vi "Autopatcher Daemon.vi"(0 "Controls":T8, 1 "Break in Thr [MOhm]":refnum<vi>, 2 "Detection Thr [%]":refnum<vi>, 3 "Disengage Target":refnum<vi>, 4 "Manipulator Dynamics":refnum<vi>, 5 "Unblockage Parameters":T7, 6 "Sensed Resistance Levels":T4, 7 "Error In":errorcluster, 8 "Signals":T9, 9 "Pressure Controls":T11, 10 "Holding Potential Controls":T2, 11 "Autotune Gain":T3, 12 "Calibration levels":T6, 13 "Manipulator Controllers":T10, 14 "Capacitance Compensation":refnum<vi>, 15 "Test and Offset Controls":T5, 16 "Dialog Indicator":refnum<vi>, 17 "Seal Dynamics":T1, 18 "Reset":refnum<vi>, 19 "Manipulator Transformation Matrix":refnum<vi>, 20 "State":refnum<vi>) -> (27 "Error Out":errorcluster)   [LabVIEW 2012, in "Autopatcher Daemon.lvlib"]
uses:
  Autopatcher Daemon.lvlib
  <vilib>/Analysis/Matrix/Datatypes/RealMatrix.ctl
  State.ctl
  <vilib>/Analysis/Matrix/NI_Matrix.lvlib
panel:
  out "Abort":refnum<vi>
  out "Exit":bool
  in  "Period":u32=100
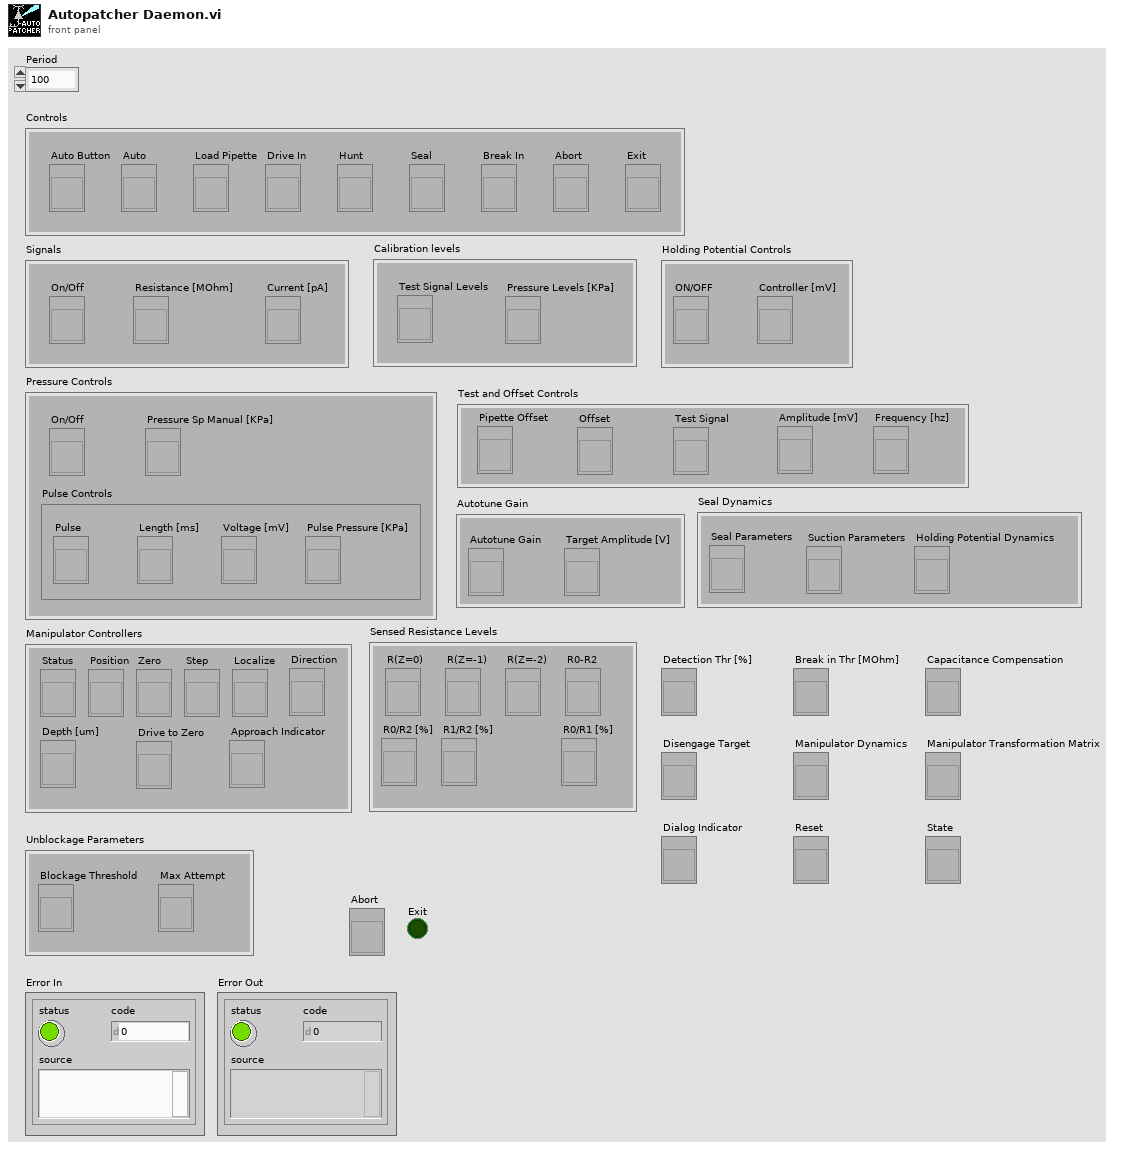
[diagram p1: front panel]
types:
  T1 = cluster{"Suction Parameters":refnum<vi>, "Holding Potential Dynamics":refnum<vi>, "Seal Parameters":refnum<vi>}
  T2 = cluster{"ON/OFF":refnum<vi>, "Controller [mV]":refnum<vi>}
  T3 = cluster{"Autotune Gain":refnum<vi>, "Target Amplitude [V]":refnum<vi>}
  T4 = cluster{"R(Z=0)":refnum<vi>, "R(Z=-1)":refnum<vi>, "R(Z=-2)":refnum<vi>, "R0-R2":refnum<vi>, "R0/R2 [%]":refnum<vi>, "R1/R2 [%]":refnum<vi>, "R0/R1 [%]":refnum<vi>}
  T5 = cluster{"Pipette Offset":refnum<vi>, "Offset":refnum<vi>, "Test Signal":refnum<vi>, "Amplitude [mV]":refnum<vi>, "Frequency [hz]":refnum<vi>}
  T6 = cluster{"Test Signal Levels":refnum<vi>, "Pressure Levels [KPa]":refnum<vi>}
  T7 = cluster{"Blockage Threshold":refnum<vi>, "Max Attempt":refnum<vi>}
  T8 = cluster{"Load Pipette":refnum<vi>, "Drive In":refnum<vi>, "Hunt":refnum<vi>, "Seal":refnum<vi>, "Break In":refnum<vi>, "Abort":refnum<vi>, "Exit":refnum<vi>, "Auto":refnum<vi>, "Auto Button":refnum<vi>}
  T9 = cluster{"On/Off":refnum<vi>, "Resistance [MOhm]":refnum<vi>, "Current [pA]":refnum<vi>}
  T10 = cluster{"Status":refnum<vi>, "Position":refnum<vi>, "Zero":refnum<vi>, "Step":refnum<vi>, "Localize":refnum<vi>, "Approach Indicator":refnum<vi>, "Depth [um]":refnum<vi>, "Drive to Zero":refnum<vi>, "Direction":refnum<vi>}
  T11 = cluster{"On/Off":refnum<vi>, "Pulse Controls":cluster{"Pulse":refnum<vi>, "Length [ms]":refnum<vi>, "Voltage [mV]":refnum<vi>, "Pulse Pressure [KPa]":refnum<vi>}, "Pressure Sp Manual [KPa]":refnum<vi>}
  T12 = typedef "State.ctl" = enum16{"READY", "LOAD", "LOCALIZATION", "HUNTING", "SEAL", "BREAKIN", "WCR", "ALIGN", "APPROACH", "TARGETING"}
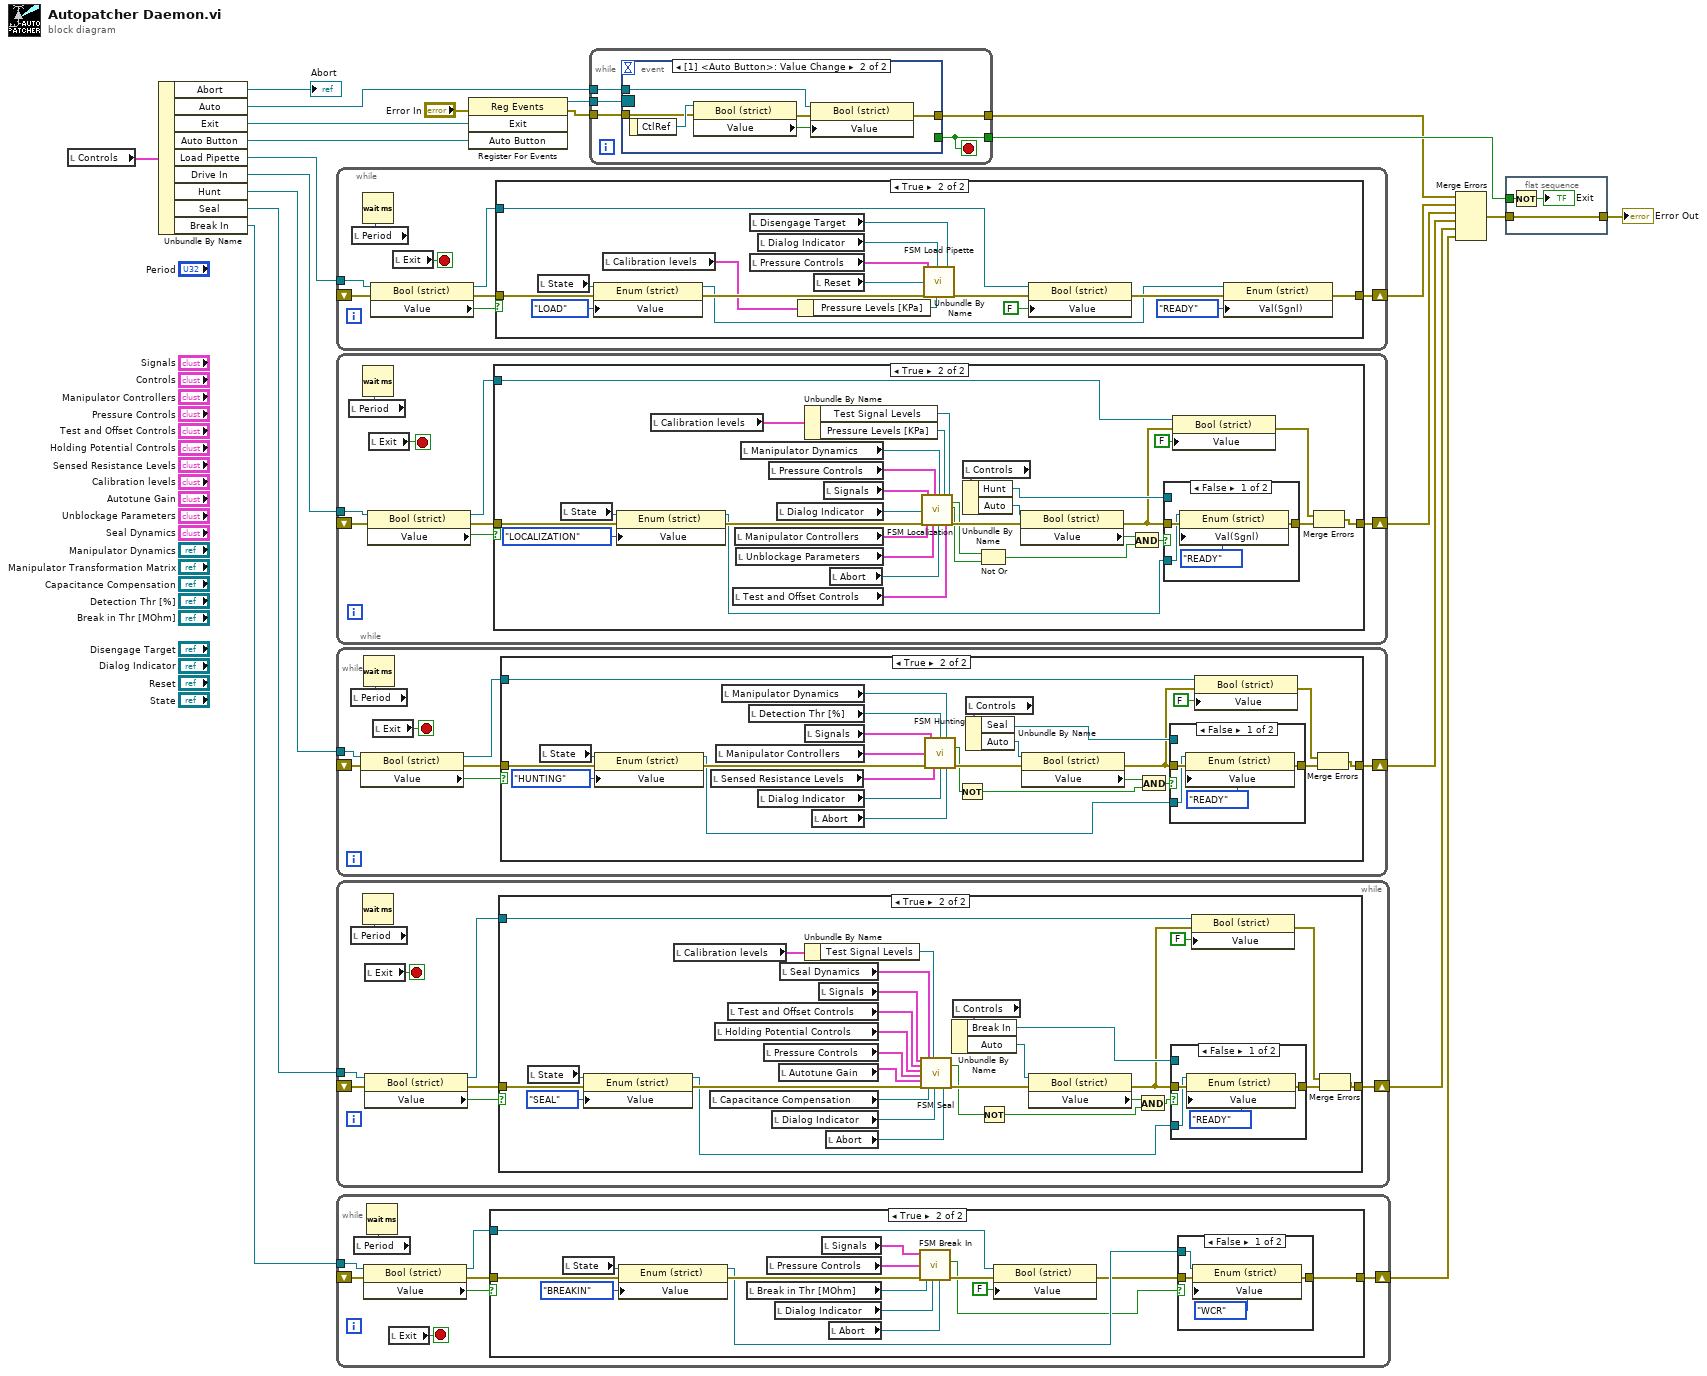
[diagram p0: block diagram]
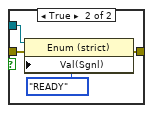
[diagram p3: hidden frame]
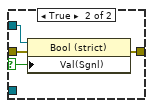
[diagram p5: hidden frame]
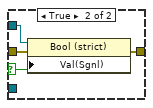
[diagram p7: hidden frame]
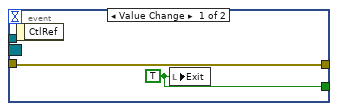
[diagram p8: hidden frame]
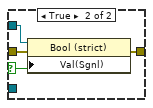
[diagram p10: hidden frame]
diagram:
  n1 = local read "Controls"() -> (w11:T8)
  n2 = Unbundle By Name(w11) -> ("Abort"=→"Abort":refnum<vi>, "Auto"=w3:refnum<vi>, "Exit"=w6:refnum<vi>, "Auto Button"=w5:refnum<vi>, "Load Pipette"=w16:refnum<vi>, "Drive In"=w15:refnum<vi>, "Hunt"=w13:refnum<vi>, "Seal"=w12:refnum<vi>, "Break In"=w10:refnum<vi>)
  n3 = while {
    tunnel: w16 -> [w30]
    shift-right: [w25] -> w21
    shift-left: _ -> [w23]
    stop <- w26 stop-if-true
    n4 = local read "Period"() -> (w27:u32)
    n5 = Wait (ms)(milliseconds to wait=w27) -> ()  [unwired: 1 out]
    n6 = property class="Bool (strict)"(reference=w30, error in=w23) -> (reference out=w24:refnum<vi>, error out=w28:errorcluster, "Value"=w29:bool)
    n7 = local read "Exit"() -> (w26:bool)
    n8 = case shown="True" w29 {
      tunnel: w28 -> [w31 w35]
      tunnel: [w31 w41] -> w25
      tunnel: w24 -> [_ w39]
      frame False {
      }
      frame True {
        n9 = local read "State"() -> (w38:refnum<vi>)
        n10 = property class="Enum (strict)"(reference=w38, error in=w35, "Value"=State."LOAD") -> (reference out=w34:refnum<vi>, error out=w36:errorcluster)
        n11 = local read "Calibration levels"() -> (w32:T6)
        n12 = local read "Disengage Target"() -> (w46:refnum<vi>)
        n13 = local read "Pressure Controls"() -> (w48:T11)
        n14 = local read "Dialog Indicator"() -> (w47:refnum<vi>)
        n15 = Unbundle By Name(w32) -> ("Pressure Levels [KPa]"=w33:refnum<vi>)
        n16 = local read "Reset"() -> (w45:refnum<vi>)
        n17 = call "FSM Load Pipette.vi"("Dialog Indicator"=w47, "Pressure Controls"=w48, "Reset"=w45, "error in (no error)"=w36, "Disengage Target"=w46, "Pressure Levels [KPa]"=w33) -> ("error out"=w40:errorcluster)  [unwired: 13 in]
        n18 = property class="Bool (strict)"(reference=w39, error in=w40, "Value"=FALSE) -> (error out=w42:errorcluster)  [unwired: 1 out]
        n19 = property class="Enum (strict)"(reference=w34, error in=w42, "Val(Sgnl)"=State."READY" ("Value")) -> (error out=w41:errorcluster)  [unwired: 1 out]
      }
    }
  }
  n20 = while {
    tunnel: w15 -> [w56]
    shift-right: [w50] -> w20
    shift-left: _ -> [w49]
    stop <- w52 stop-if-true
    n21 = local read "Period"() -> (w53:u32)
    n22 = Wait (ms)(milliseconds to wait=w53) -> ()  [unwired: 1 out]
    n23 = property class="Bool (strict)"(reference=w56, error in=w49) -> (reference out=w51:refnum<vi>, error out=w54:errorcluster, "Value"=w55:bool)
    n24 = local read "Exit"() -> (w52:bool)
    n25 = case shown="True" w55 {
      tunnel: w54 -> [w57 w65]
      tunnel: [w57 w71] -> w50
      tunnel: w51 -> [_ w72]
      frame False {
      }
      frame True {
        n26 = local read "State"() -> (w67:refnum<vi>)
        n27 = property class="Enum (strict)"(reference=w67, error in=w65, "Value"=State."LOCALIZATION") -> (reference out=w61:refnum<vi>, error out=w66:errorcluster)
        n28 = local read "Calibration levels"() -> (w82:T6)
        n29 = local read "Test and Offset Controls"() -> (w80:T5)
        n30 = local read "Manipulator Controllers"() -> (w87:T10)
        n31 = local read "Unblockage Parameters"() -> (w83:T7)
        n32 = local read "Manipulator Dynamics"() -> (w88:refnum<vi>)
        n33 = local read "Pressure Controls"() -> (w86:T11)
        n34 = local read "Dialog Indicator"() -> (w79:refnum<vi>)
        n35 = Unbundle By Name(w82) -> ("Test Signal Levels"=w78:refnum<vi>, "Pressure Levels [KPa]"=w81:refnum<vi>)
        n36 = local read "Signals"() -> (w85:T9)
        n37 = local read "Abort"() -> (w84:refnum<vi>)
        n38 = call "FSM Localization.vi"("Signals"=w85, "Pressure Controls"=w86, "Dialog Indicator"=w79, "error in (no error)"=w66, "Manipulator Dynamics"=w88, "Unblockage Parameters"=w83, "Pressure Levels [KPa]"=w81, "Test and Offset Controls"=w80, "Test Signal Levels"=w78, "Manipulator Controllers"=w87, "Abort"=w84) -> ("Aborted"=w59:bool, "Blocked"=w60:bool, "error out"=w75:errorcluster)  [unwired: 6 in]
        n39 = local read "Controls"() -> (w76:T8)
        n40 = Unbundle By Name(w76) -> ("Hunt"=w74:refnum<vi>, "Auto"=w77:refnum<vi>)
        n41 = Not Or(1:w60, 2:w59) -> (0:w58:bool)
        n42 = property class="Bool (strict)"(reference=w77, error in=w75) -> (error out=w64:errorcluster, "Value"=w62:bool)  [unwired: 1 out]
        n43 = And(x=w62, y=w58) -> (x .and. y?=w63:bool)
        n44 = case shown="False" w63 {
          selector: w63 -> [_ w94]
          tunnel: w64 -> [w92 w96]
          tunnel: w74 -> [_ w95]
          tunnel: [w91 w93] -> w70
          tunnel: w61 -> [w90 _]
          frame False {
            n45 = property class="Enum (strict)"(reference=w90, error in=w92, "Val(Sgnl)"=State."READY" ("Value")) -> (error out=w91:errorcluster)  [unwired: 1 out]
          }
          frame True {
            n46 = property class="Bool (strict)"(reference=w95, error in=w96, "Val(Sgnl)"=w94) -> (error out=w93:errorcluster)  [unwired: 1 out]
          }
        }
        n47 = property class="Bool (strict)"(reference=w72, error in=w64, "Value"=FALSE) -> (error out=w69:errorcluster)  [unwired: 1 out]
        n48 = Merge Errors(w69, w70) -> (w71:errorcluster)
      }
    }
  }
  n49 = while {
    tunnel: w13 -> [w104]
    shift-right: [w98] -> w9
    shift-left: _ -> [w97]
    stop <- w102 stop-if-true
    n50 = local read "Period"() -> (w100:u32)
    n51 = property class="Bool (strict)"(reference=w104, error in=w97) -> (reference out=w99:refnum<vi>, error out=w101:errorcluster, "Value"=w103:bool)
    n52 = Wait (ms)(milliseconds to wait=w100) -> ()  [unwired: 1 out]
    n53 = local read "Exit"() -> (w102:bool)
    n54 = case shown="True" w103 {
      tunnel: w101 -> [w105 w113]
      tunnel: [w105 w117] -> w98
      tunnel: w99 -> [_ w124]
      frame False {
      }
      frame True {
        n55 = local read "State"() -> (w115:refnum<vi>)
        n56 = property class="Enum (strict)"(reference=w115, error in=w113, "Value"=State."HUNTING") -> (reference out=w106:refnum<vi>, error out=w114:errorcluster)
        n57 = local read "Sensed Resistance Levels"() -> (w126:T4)
        n58 = local read "Manipulator Controllers"() -> (w131:T10)
        n59 = local read "Manipulator Dynamics"() -> (w129:refnum<vi>)
        n60 = local read "Detection Thr [%]"() -> (w127:refnum<vi>)
        n61 = local read "Dialog Indicator"() -> (w128:refnum<vi>)
        n62 = local read "Signals"() -> (w130:T9)
        n63 = local read "Abort"() -> (w107:refnum<vi>)
        n64 = call "FSM Hunting.vi"("Signals"=w130, "Detection Thr [%]"=w127, "Manipulator Dynamics"=w129, "Manipulator Controllers"=w131, "Sensed Resistance Levels"=w126, "error in (no error)"=w114, "Dialog Indicator"=w128, "Abort"=w107) -> ("Aborted"=w111:bool, "error out"=w119:errorcluster)  [unwired: 6 in]
        n65 = Not(x=w111) -> (.not. x?=w108:bool)
        n66 = local read "Controls"() -> (w121:T8)
        n67 = Unbundle By Name(w121) -> ("Seal"=w123:refnum<vi>, "Auto"=w122:refnum<vi>)
        n68 = property class="Bool (strict)"(reference=w122, error in=w119) -> (error out=w112:errorcluster, "Value"=w110:bool)  [unwired: 1 out]
        n69 = And(x=w110, y=w108) -> (x .and. y?=w109:bool)
        n70 = case shown="False" w109 {
          selector: w109 -> [_ w137]
          tunnel: w112 -> [w134 w139]
          tunnel: w123 -> [_ w138]
          tunnel: [w135 w136] -> w120
          tunnel: w106 -> [w133 _]
          frame False {
            n71 = property class="Enum (strict)"(reference=w133, error in=w134, "Value"=State."READY") -> (error out=w135:errorcluster)  [unwired: 1 out]
          }
          frame True {
            n72 = property class="Bool (strict)"(reference=w138, error in=w139, "Val(Sgnl)"=w137) -> (error out=w136:errorcluster)  [unwired: 1 out]
          }
        }
        n73 = property class="Bool (strict)"(reference=w124, error in=w112, "Value"=FALSE) -> (error out=w118:errorcluster)  [unwired: 1 out]
        n74 = Merge Errors(w118, w120) -> (w117:errorcluster)
      }
    }
  }
  n75 = while {
    tunnel: w12 -> [w141]
    shift-right: [w142] -> w8
    shift-left: _ -> [w140]
    stop <- w146 stop-if-true
    n76 = local read "Period"() -> (w144:u32)
    n77 = Wait (ms)(milliseconds to wait=w144) -> ()  [unwired: 1 out]
    n78 = local read "Exit"() -> (w146:bool)
    n79 = property class="Bool (strict)"(reference=w141, error in=w140) -> (reference out=w143:refnum<vi>, error out=w145:errorcluster, "Value"=w147:bool)
    n80 = case shown="True" w147 {
      tunnel: w145 -> [w148 w155]
      tunnel: [w148 w159] -> w142
      tunnel: w143 -> [_ w161]
      frame False {
      }
      frame True {
        n81 = local read "State"() -> (w157:refnum<vi>)
        n82 = property class="Enum (strict)"(reference=w157, error in=w155, "Value"=State."SEAL") -> (reference out=w149:refnum<vi>, error out=w156:errorcluster)
        n83 = local read "Calibration levels"() -> (w178:T6)
        n84 = local read "Capacitance Compensation"() -> (w168:refnum<vi>)
        n85 = local read "Holding Potential Controls"() -> (w170:T2)
        n86 = local read "Test and Offset Controls"() -> (w171:T5)
        n87 = local read "Pressure Controls"() -> (w174:T11)
        n88 = local read "Dialog Indicator"() -> (w176:refnum<vi>)
        n89 = local read "Autotune Gain"() -> (w175:T3)
        n90 = local read "Seal Dynamics"() -> (w169:T1)
        n91 = Unbundle By Name(w178) -> ("Test Signal Levels"=w173:refnum<vi>)
        n92 = local read "Signals"() -> (w172:T9)
        n93 = local read "Abort"() -> (w177:refnum<vi>)
        n94 = call "FSM Seal.vi"("Signals"=w172, "Test and Offset Controls"=w171, "Holding Potential Controls"=w170, "Pressure Controls"=w174, "Autotune Gain"=w175, "error in (no error)"=w156, "Seal Dynamics"=w169, "Capacitance Compensation"=w168, "Test Signal Levels"=w173, "Dialog Indicator"=w176, "Abort"=w177) -> ("Aborted"=w151:bool, "error out"=w163:errorcluster)  [unwired: 7 in]
        n95 = local read "Controls"() -> (w165:T8)
        n96 = Unbundle By Name(w165) -> ("Break In"=w162:refnum<vi>, "Auto"=w166:refnum<vi>)
        n97 = Not(x=w151) -> (.not. x?=w150:bool)
        n98 = property class="Bool (strict)"(reference=w166, error in=w163) -> (error out=w154:errorcluster, "Value"=w152:bool)  [unwired: 1 out]
        n99 = And(x=w152, y=w150) -> (x .and. y?=w153:bool)
        n100 = case shown="False" w153 {
          selector: w153 -> [_ w184]
          tunnel: w154 -> [w181 w186]
          tunnel: w162 -> [_ w185]
          tunnel: [w182 w183] -> w164
          tunnel: w149 -> [w180 _]
          frame False {
            n101 = property class="Enum (strict)"(reference=w180, error in=w181, "Value"=State."READY") -> (error out=w182:errorcluster)  [unwired: 1 out]
          }
          frame True {
            n102 = property class="Bool (strict)"(reference=w185, error in=w186, "Val(Sgnl)"=w184) -> (error out=w183:errorcluster)  [unwired: 1 out]
          }
        }
        n103 = property class="Bool (strict)"(reference=w161, error in=w154, "Value"=FALSE) -> (error out=w160:errorcluster)  [unwired: 1 out]
        n104 = Merge Errors(w160, w164) -> (w159:errorcluster)
      }
    }
  }
  n105 = while {
    tunnel: w10 -> [w194]
    shift-right: [w189] -> w7
    shift-left: _ -> [w187]
    stop <- w192 stop-if-true
    n106 = local read "Period"() -> (w190:u32)
    n107 = property class="Bool (strict)"(reference=w194, error in=w187) -> (reference out=w188:refnum<vi>, error out=w191:errorcluster, "Value"=w193:bool)
    n108 = Wait (ms)(milliseconds to wait=w190) -> ()  [unwired: 1 out]
    n109 = local read "Exit"() -> (w192:bool)
    n110 = case shown="True" w193 {
      tunnel: w191 -> [w195 w201]
      tunnel: [w195 w199] -> w189
      tunnel: w188 -> [_ w205]
      frame False {
      }
      frame True {
        n111 = local read "State"() -> (w204:refnum<vi>)
        n112 = property class="Enum (strict)"(reference=w204, error in=w201, "Value"=State."BREAKIN") -> (reference out=w198:refnum<vi>, error out=w202:errorcluster)
        n113 = local read "Break in Thr [MOhm]"() -> (w208:refnum<vi>)
        n114 = local read "Pressure Controls"() -> (w209:T11)
        n115 = local read "Dialog Indicator"() -> (w207:refnum<vi>)
        n116 = local read "Signals"() -> (w210:T9)
        n117 = local read "Abort"() -> (w211:refnum<vi>)
        n118 = call "FSM Break In.vi"("Abort"=w211, "Dialog Indicator"=w207, "error in (no error)"=w202, "Break in Thr [MOhm]"=w208, "Pressure Controls"=w209, "Signals"=w210) -> ("error out"=w206:errorcluster, "Aborted"=w196:bool)  [unwired: 4 in]
        n119 = property class="Bool (strict)"(reference=w205, error in=w206, "Value"=FALSE) -> (error out=w197:errorcluster)  [unwired: 1 out]
        n120 = case shown="False" w196 {
          tunnel: w198 -> [w214 w219]
          tunnel: [w212 w218] -> w199
          tunnel: w197 -> [w213 w217]
          frame False {
            n121 = property class="Enum (strict)"(reference=w214, error in=w213, "Value"=State."WCR") -> (error out=w212:errorcluster)  [unwired: 1 out]
          }
          frame True {
            n122 = property class="Enum (strict)"(reference=w219, error in=w217, "Val(Sgnl)"=State."READY" ("Value")) -> (error out=w218:errorcluster)  [unwired: 1 out]
          }
        }
      }
    }
  }
  n123 = register-events(error in="Error In", w6, w5) -> (reference out=w22:refnum<event-registration>, error out=w2:errorcluster)  [unwired: 1 in]
  n124 = while {
    tunnel: w22 -> [w224]
    tunnel: [w223] -> w17
    tunnel: w3 -> [w222]
    tunnel: w2 -> [w221]
    tunnel: [w220] -> w1
    stop <- w223 stop-if-true
    n125 = event shown="[1] <Auto Button>: Value Change" {
      selector: w224 -> [_ _]
      dyn-events: _ -> [_ _]
      timeout: _ -> [_ _]
      tunnel: [w226 _] -> w223
      tunnel: w222 -> [_ w229]
      tunnel: w221 -> [w225 w228]
      tunnel: [w225 w227] -> w220
      event Value Change {
        w226 = TRUE ("Exit")
        n126 = event-data() -> ()  [unwired: 1 in, 1 out]
        n127 = local write "Exit"(w226) -> ()
      }
      event Value Change {
        n128 = event-data() -> ("CtlRef"=w232:refnum<vi>)  [unwired: 1 in]
        n129 = property class="Bool (strict)"(reference=w232, error in=w228) -> (error out=w230:errorcluster, "Value"=w231:bool)  [unwired: 1 out]
        n130 = property class="Bool (strict)"(reference=w229, error in=w230, "Value"=w231) -> (error out=w227:errorcluster)  [unwired: 1 out]
      }
    }
  }
  n131 = Merge Errors(w1, w21, w20, w9, w8, w7) -> (w19:errorcluster)
  n132 = flat-sequence {
    tunnel: [w235] -> w18
    tunnel: w19 -> [w235]
    tunnel: w17 -> [w234]
    frame #0 {
      n133 = Not(x=w234) -> (.not. x?=→"Exit":bool)
    }
  }
  "Error Out" <- w18
